vi "Configure Math Expression (Unary Operation).vi"(7 "Operator (0: AVG)":u16(ring) items=["AVG", "SQRT", "FABS", "Integral", "Log10", "Ceil", "Derivative", "LogE", "Floor", "Invert", "Exp", "Sin", "Cos", "Tan", "ASin", "ACos", "ATan", "Sinh", "Cosh", "Tanh", "Min", "Max", "wfmDB", "Spectral Mag", "Spectral Real", "Spectral Phase", "Spectral Imaginary"], 8 "error in (no error)":errorcluster, 10 "Expression Input 1":string(combo), 11 "VISA resource name":refnum<visa-resource-name>) -> (0 "error out":errorcluster, 2 "Expression Output":string, 3 "VISA resource name out":refnum<visa-resource-name>)   [LabVIEW 2015, in "Tektronix 7000 Series.lvlib"]
doc: "Creates a mathematical expression with one operand.\n\n<B>Note:</B> The TDS 5000 series will not support most unary functions or support nested functions without the math option installed."
uses:
  <instrlib>/Tektronix 7000 Series/Tektronix 7000 Series.lvlib
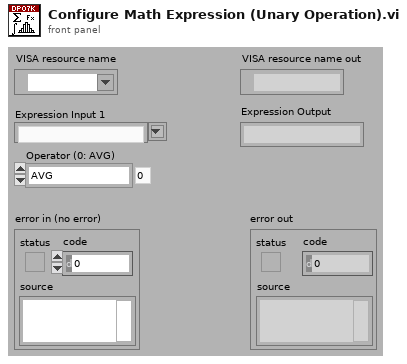
[diagram p1: front panel]
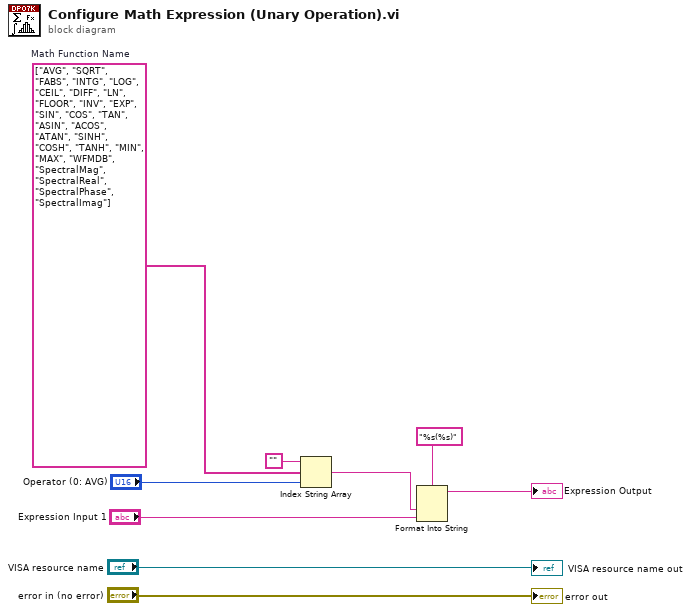
[diagram p0: block diagram]
diagram:
  w6 = string[] ["AVG", "SQRT", "FABS", "INTG", "LOG", "CEIL", "DIFF", "LN", "FLOOR", "INV", "EXP", "SIN", "COS", "TAN", "ASIN", "ACOS", "ATAN", "SINH", "COSH", "TANH", "MIN", "MAX", "WFMDB", "SpectralMag", "SpectralReal", "SpectralPhase", "SpectralImag"]  # Math Function Name
  n1 = Index String Array(1:"Operator (0: AVG)", 2:w6, 3:"" ("Empty String Constant")) -> (0:w4:string)
  n2 = Format Into String(format string="%s(%s)", w4, "Expression Input 1") -> (resulting string=→"Expression Output":string)  [unwired: 2 in, 1 out]
  "VISA resource name out" <- "VISA resource name"
  "error out" <- "error in (no error)"
